vi "a2i.vi"() -> ()   [LabVIEW 2022 SP3]
panel:
  in  "Failed program":bool
  in  "Pass program":bool
  in  "Take program":bool
  out "Request processed":bool
  out "Passed":bool
  out "Taking program":bool
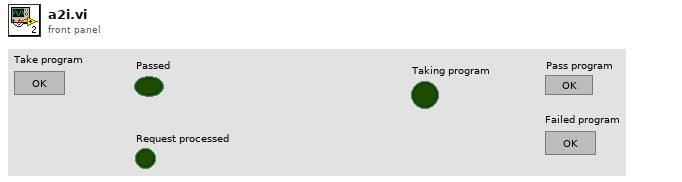
[diagram p1: front panel]
types:
  T1 = enum16{"Start", "Taking Program", "Passed", "Failed"}
  T2 = enum16{"Start", "Taking Program", "Passed", "Failed", ""}
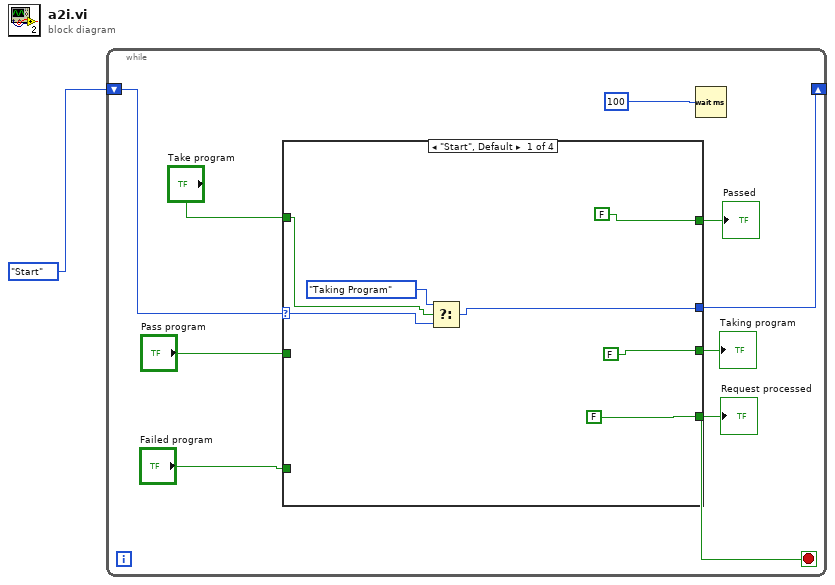
[diagram p0: block diagram]
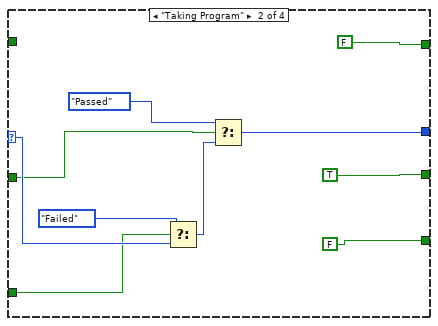
[diagram p2: hidden frame]
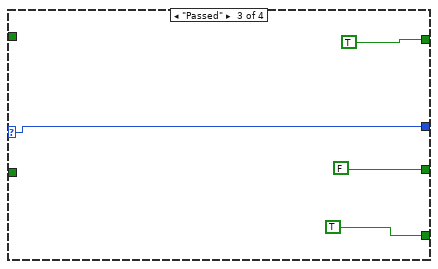
[diagram p3: hidden frame]
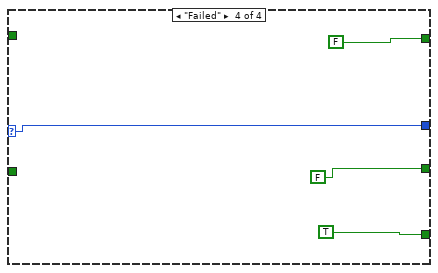
[diagram p4: hidden frame]
diagram:
  n1 = while {
    shift-right: [w10] -> _
    shift-left: T1."Start" -> [w9]
    stop <- w6 stop-if-true
    n2 = case shown="\"Start\", Default" w9 {
      selector: w9 -> [w16 w26 w28 w32]
      tunnel: [w15 w23 w28 w32] -> w10
      tunnel: [FALSE TRUE FALSE FALSE] -> w7
      tunnel: "Failed program" -> [_ w21 _ _]
      tunnel: "Pass program" -> [_ w18 _ _]
      tunnel: [FALSE FALSE TRUE TRUE] -> w6
      tunnel: [FALSE FALSE TRUE FALSE] -> w8
      tunnel: "Take program" -> [w11 _ _ _]
      frame "Start", Default {
        n3 = Select(t=T2."Taking Program", s=w11, f=w16) -> (s? t:f=w15:T2)
      }
      frame "Taking Program" {
        n4 = Select(t=T1."Failed", s=w21, f=w26) -> (s? t:f=w24:T2)
        n5 = Select(t=T1."Passed", s=w18, f=w24) -> (s? t:f=w23:T2)
      }
      frame "Passed" {
      }
      frame "Failed" {
      }
    }
    "Request processed" <- w6
    "Taking program" <- w7
    "Passed" <- w8
    n6 = Wait (ms)(milliseconds to wait=100) -> ()  [unwired: 1 out]
  }
